vi "SlidingTraces.vi"(1 "sliding traces in":T1(array[cluster]) {"SlideCenterPeak" format="%.2f"; "SlideTime" format="%.2f"}, 2 "set":bool) -> (0 "sliding traces out":T1(array[cluster]) {"SlideCenterPeak" format="%.2f"; "SlideTime" format="%.2f"})   [LabVIEW 2009]
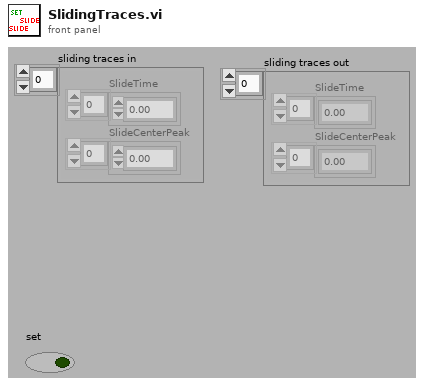
[diagram p1: front panel]
types:
  T1 = cluster{"SlideTime":dbl[], "SlideCenterPeak":dbl[]}[]
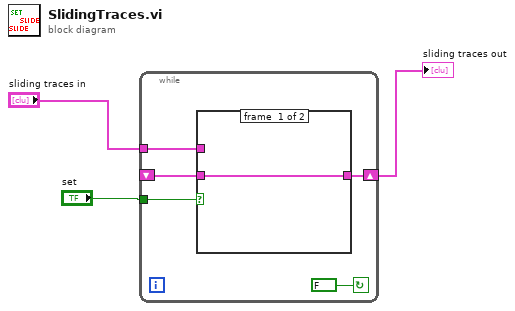
[diagram p0: block diagram]
diagram:
  n1 = while {
    shift-right: [w6] -> w1
    shift-left: _ -> [w4]
    tunnel: "set" -> [w7]
    tunnel: "sliding traces in" -> [w5]
    stop <- FALSE continue-if-true
    n2 = case shown="True" w7 {
      tunnel: [w9 w10] -> w6
      tunnel: w5 -> [_ w10]
      tunnel: w4 -> [w9 _]
      frame #0 {
      }
      frame #1 {
      }
    }
  }
  "sliding traces out" <- w1
